vi "CRYFFT CRYSoundLab.vi"(9 "dt":dbl=2.2675737e-05 format="%.7e", 10 "Window":i32(ring)=1 items=["None (Uniform)", "Hanning", "Hamming", "Blackman-Harris", "Exact Blackman", "Blackman", "Flat Top", "4 Term B-Harris", "7 Term B-Harris"], 11 "Time series":dbl[](array[numeric]) format="%.2f") -> (1 "window constants":cluster{"eq noise BW":dbl, "coherent gain":dbl} {"coherent gain" format="%.2f"; "eq noise BW" format="%.2f"}, 2 "df":dbl format="%.2f", 3 "Power Spectrum (V^2 rms)":dbl[](array[numeric]) format="%.2f")   [LabVIEW 2013]
uses:
  <vilib>/Analysis/0measdsp.llb/Scaled Time Domain Window (DBL).vi
  <vilib>/Analysis/NI_AALPro.lvlib
panel:
  out "size(s)":i32
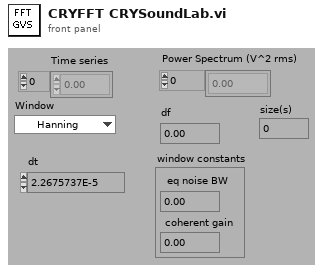
[diagram p1: front panel]
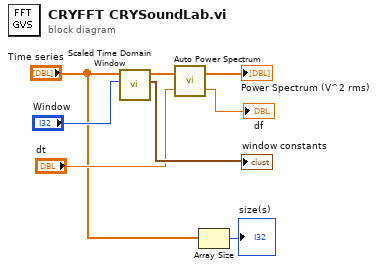
[diagram p0: block diagram]
diagram:
  n1 = call-poly <vilib>:"Scaled Time Domain Window.vi"("window"="Window", "X"="Time series") -> ("window properties"=→"window constants":cluster{"eq noise BW":dbl, "coherent gain":dbl}, "Windowed X"=w8:dbl[])  [unwired: 1 in, 7 out]
  n2 = call <vilib>:"Auto Power Spectrum.vi"("dt"="dt", "Signal (V)"=w8) -> ("df"=→"df":dbl, "Power Spectrum (V^2 rms)"=→"Power Spectrum (V^2 rms)":dbl[])
  n3 = Array Size(array="Time series") -> (size(s)=→"size(s)":i32)
